vi "Static Error Handling.Static String.vi"   [LabVIEW 2016, in "Memory Manager.lvlib" / "Static Error Handling.lvlib"]
uses:
  Static Error Handling.lvlib
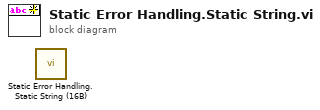
[diagram p0: block diagram]
diagram:
  n1 = call "Static Error Handling.Static String (16B).vi"() -> ()  [unwired: 11 in, 1 out]
